vi "getTopMostBlockDiagram.vi"(6 "closeAppRef":bool=TRUE, 8 "error in (no error)":errorcluster, 11 "appReference":refnum<vi>) -> (0 "error out":errorcluster, 3 "topMostBlockDiagram":refnum<class "BlockDiagram.lvclass">)   [LabVIEW 2023, in "TLC_Scripto.lvlib"]
uses:
  TLC_Scripto.lvlib
  BlockDiagram/BlockDiagram.lvclass
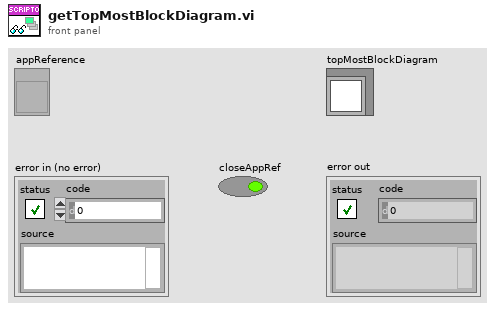
[diagram p1: front panel]
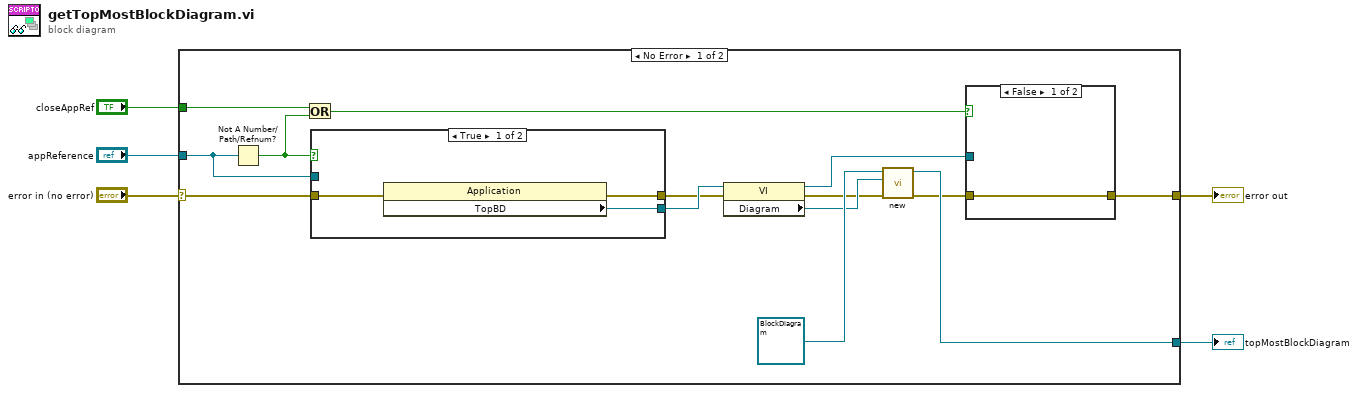
[diagram p0: block diagram]
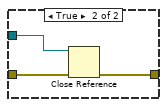
[diagram p2: hidden frame]
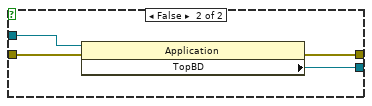
[diagram p3: hidden frame]
diagram:
  n1 = case shown="No Error" "error in (no error)" {
    selector: "error in (no error)" -> [w18 w31]
    tunnel: "appReference" -> [w19 _]
    tunnel: [w14 _] -> w2
    tunnel: [w12 w31] -> w3
    tunnel: "closeAppRef" -> [w6 _]
    frame No Error {
      n2 = Not A Number/Path/Refnum?(number/path/refnum=w19) -> (NaN/Path/Refnum?=w8:bool)
      n3 = Or(x=w6, y=w8) -> (x .or. y?=w7:bool)
      n4 = case shown="True" w8 {
        tunnel: [w26 w30] -> w10
        tunnel: w18 -> [w25 w29]
        tunnel: w19 -> [_ w28]
        tunnel: [w24 w27] -> w9
        frame True {
          n5 = property class="Application"(error in=w25) -> (error out=w24:errorcluster, "TopBD"=w26:refnum<vi>)  [unwired: 1 in, 1 out]
        }
        frame False {
          n6 = property class="Application"(reference=w28, error in=w29) -> (error out=w27:errorcluster, "TopBD"=w30:refnum<vi>)  [unwired: 1 out]
        }
      }
      n7 = property class="VI"(reference=w10, error in=w9) -> (reference out=w11:refnum<vi>, error out=w15:errorcluster, "Diagram"=w16:refnum<vi>)
      n8 = call-dynamic "new.vi"("Error In"=w15, "ref"=w16, "GObject in"=refnum<class "BlockDiagram.lvclass"> refnum ("TLC_Scripto.lvlib:BlockDiagram.lvclass")) -> ("Error Out"=w13:errorcluster, "GObject out"=w14:refnum<class "BlockDiagram.lvclass">)  [unwired: 7 in]
      n9 = case shown="False" w7 {
        tunnel: w13 -> [w20 w23]
        tunnel: [w20 w22] -> w12
        tunnel: w11 -> [_ w21]
        frame False {
        }
        frame True {
          n10 = Close Reference(reference=w21, error in (no error)=w23) -> (error out=w22:errorcluster)
        }
      }
    }
    frame Error {
    }
  }
  "error out" <- w3
  "topMostBlockDiagram" <- w2
